vi "Create Variant Dictionary.vi"(7 "SMO.Dictionary.Variant":refnum<class "SMO.Dictionary.Variant.lvclass">, 8 "error in (no error)":errorcluster, 10 "Subsystem Name (optional)":string) -> (0 "error out":errorcluster, 2 "SMO name":string, 3 "SMO.Dictionary.Variant out":refnum<class "SMO.Dictionary.Variant.lvclass">)   [LabVIEW 2013, in "SMO.Dictionary.lvlib" / "SMO.Dictionary.Variant.lvclass"]
uses:
  SMO.Dictionary.Variant.lvclass
  SMO.Dictionary/SMO.Dictionary.lvclass
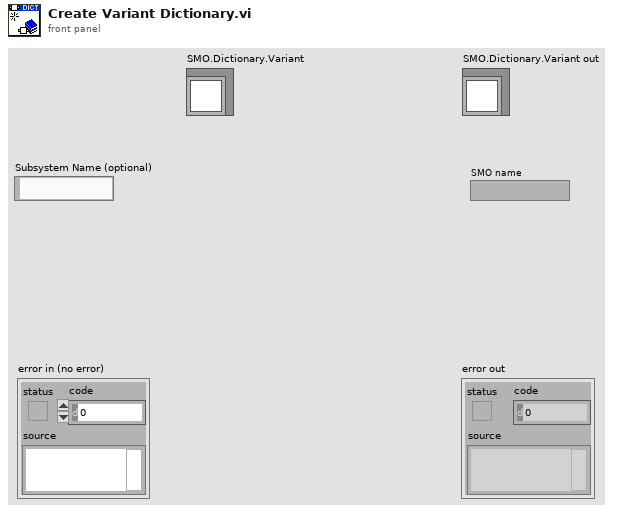
[diagram p1: front panel]
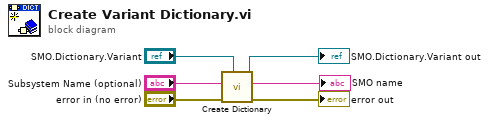
[diagram p0: block diagram]
diagram:
  n1 = call "Create Dictionary.vi"("SMO.Dictionary"="SMO.Dictionary.Variant", "error in (no error)"="error in (no error)", "Subsystem Name (optional)"="Subsystem Name (optional)") -> ("error out"=→"error out":errorcluster, "SMO name"=→"SMO name":string, "SMO.Dictionary out"=→"SMO.Dictionary.Variant out":refnum<class "SMO.Dictionary.Variant.lvclass">)  [unwired: 6 in]
